vi "timer.vi"(10 "Start/Stop":bool, 11 "Limit":dbl) -> (2 "Under limit":bool, 3 "Time elapsed":dbl)   [LabVIEW 2015]
panel:
  out "error out":errorcluster
  in  "error in (no error)":errorcluster
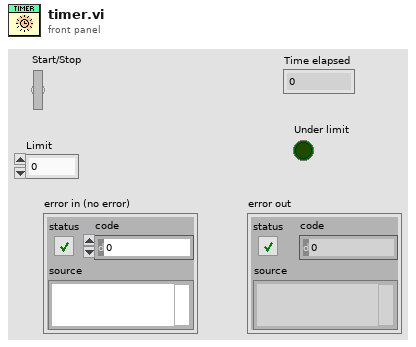
[diagram p1: front panel]
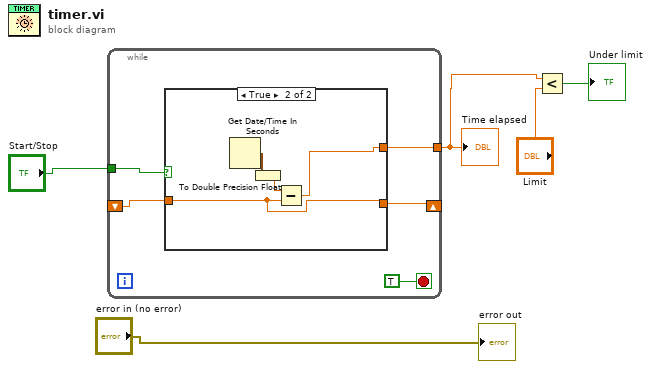
[diagram p0: block diagram]
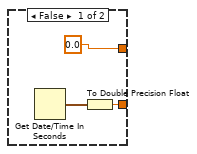
[diagram p2: hidden frame]
diagram:
  n1 = while {
    tunnel: "Start/Stop" -> [w9]
    shift-right: [w7] -> _
    shift-left: _ -> [w6]
    tunnel: [w8] -> w2
    stop <- TRUE stop-if-true
    n2 = case shown="True" w9 {
      tunnel: [0.0 w15] -> w8
      tunnel: [w11 w14] -> w7
      tunnel: w6 -> [_ w14]
      frame False {
        n3 = Get Date/Time In Seconds() -> (seconds since 1Jan1904=w12:timestamp)
        n4 = To Double Precision Float(number=w12) -> (double precision float=w11:dbl)
      }
      frame True {
        n5 = Get Date/Time In Seconds() -> (seconds since 1Jan1904=w17:timestamp)
        n6 = To Double Precision Float(number=w17) -> (double precision float=w16:dbl)
        n7 = Subtract(x=w16, y=w14) -> (x-y=w15:dbl)
      }
    }
  }
  "Time elapsed" <- w2
  n8 = Less?(x=w2, y="Limit") -> (x < y?=→"Under limit":bool)
  "error out" <- "error in (no error)"
